vi "clLabview_writeVI.vi"(0 "vi_lib.lvlib:clLabview.lvclass":refnum<class "clLabview.lvclass">, 1 "filename (use dialog)":path, 3 "new Password":string) -> (7 "vi_lib.lvlib:clLabview.lvclass [Out]":refnum<class "clLabview.lvclass">, 10 "no Error":bool)   [LabVIEW 2011, in "vi_lib.lvlib" / "clLabview.lvclass"]
uses:
  clLabview.lvclass
  clFileReader/clFileReader.lvclass
panel:
  out "MD5 password (Hex)":string
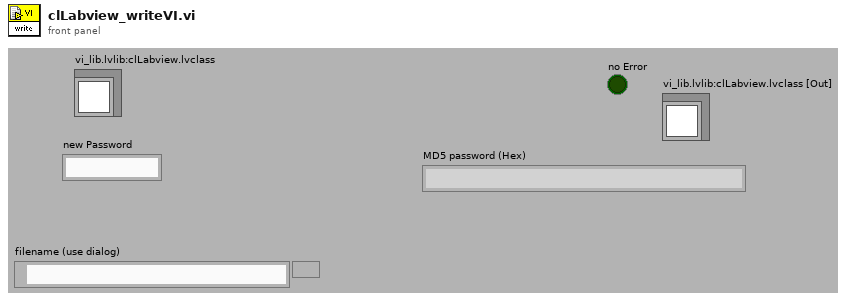
[diagram p1: front panel]
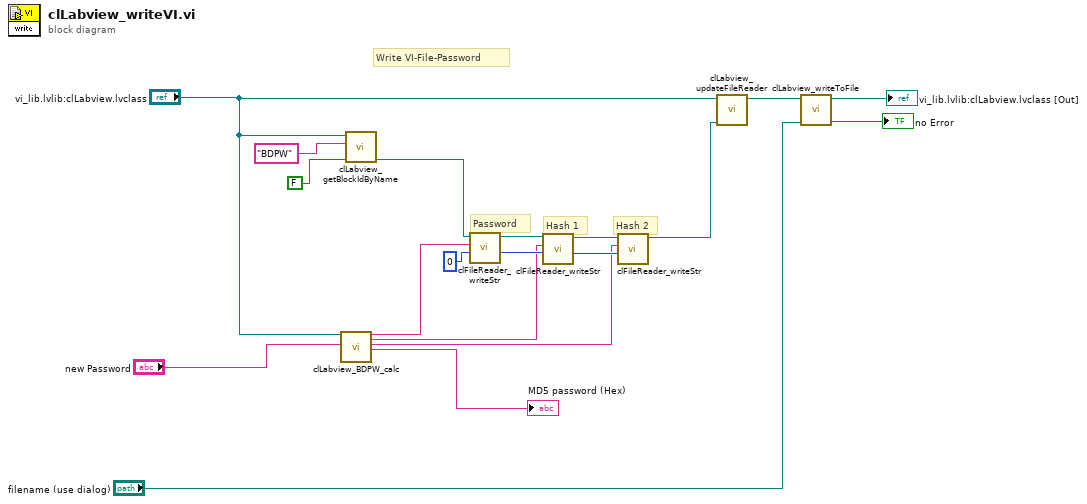
[diagram p0: block diagram]
diagram:
  # "Hash 2"
  # "Hash 1"
  # "Password"
  # "Write VI-File-Password"
  n1 = call "clLabview_BDPW_calc.vi"("vi_lib.lvlib:clLabview.lvclass"="vi_lib.lvlib:clLabview.lvclass", "new Password"="new Password") -> ("MD5 password"=w10:string, "Hash 1"=w5:string, "Hash 2"=w4:string, "MD5 password (Hex)"=→"MD5 password (Hex)":string)  [unwired: 14 out]
  n2 = call "clLabview_getBlockIdByName.vi"("use compression (off)"=FALSE, "Block Name"="BDPW", "vi_lib.lvlib:clLabview.lvclass"="vi_lib.lvlib:clLabview.lvclass") -> ("Block Content"=w3:refnum<class "clFileReader.lvclass">)  [unwired: 1 in, 6 out]
  n3 = call "clFileReader_writeStr.vi"("offset"=u32 0, "ReadStr - IN Value"=w10, "clFileReader.lvclass IN"=w3) -> ("new offset"=w8:u32, "clFileReader.lvclass OUT"=w1:refnum<class "clFileReader.lvclass">)  [unwired: 7 out]
  n4 = call "clFileReader_writeStr.vi"("offset"=w8, "ReadStr - IN Value"=w5, "clFileReader.lvclass IN"=w1) -> ("new offset"=w7:u32, "clFileReader.lvclass OUT"=w6:refnum<class "clFileReader.lvclass">)  [unwired: 7 out]
  n5 = call "clFileReader_writeStr.vi"("offset"=w7, "ReadStr - IN Value"=w4, "clFileReader.lvclass IN"=w6) -> ("clFileReader.lvclass OUT"=w19:refnum<class "clFileReader.lvclass">)  [unwired: 8 out]
  n6 = call "clLabview_updateFileReader.vi"("clFileReader.lvclass OUT"=w19, "vi_lib.lvlib:clLabview.lvclass"="vi_lib.lvlib:clLabview.lvclass") -> ("vi_lib.lvlib:clLabview.lvclass 2"=w18:refnum<class "clLabview.lvclass">)  [unwired: 9 out]
  n7 = call "clLabview_writeToFile.vi"("filename (use dialog)"="filename (use dialog)", "vi_lib.lvlib:clLabview.lvclass"=w18) -> ("no Error"=→"no Error":bool, "vi_lib.lvlib:clLabview.lvclass 2"=→"vi_lib.lvlib:clLabview.lvclass [Out]":refnum<class "clLabview.lvclass">)  [unwired: 8 out]
